vi "Read Msg Input.vi"(10 "Msg Input":refnum<class "Msg Input.lvclass">) -> (4 "Teller":refnum<class "Teller.lvclass">)   [LabVIEW 2020, in "jettl.lvlib" / "Stop jettl Msg.lvlib" / "Stop Msg Input.lvlib"]
uses:
  Stop Msg Input.lvlib
  Teller/Teller.lvclass
  Msg Input/Msg Input.lvclass
  Stop Msg Input/Stop Msg Input.lvclass
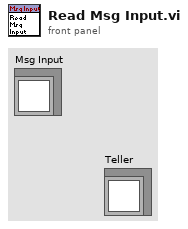
[diagram p1: front panel]
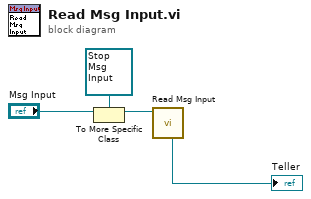
[diagram p0: block diagram]
diagram:
  n1 = To More Specific Class(target class=refnum<class "Stop Msg Input.lvclass"> refnum ("jettl.lvlib:Stop jettl Msg.lvlib:Stop Msg Input.lvlib:Stop Msg Input.lvclass"), reference="Msg Input") -> (specific class reference=w2:refnum<class "Stop Msg Input.lvclass">)  [unwired: 1 in, 1 out]
  n2 = call "Read Msg Input.vi"("Stop Msg Input in"=w2) -> ("Teller"=→"Teller":refnum<class "Teller.lvclass">)  [unwired: 10 in]
